vi "getDescription.vi"(8 "error in (no error)":errorcluster, 11 "Milk in":refnum<class "Milk.lvclass">) -> (0 "error out":errorcluster, 2 "description":string, 3 "Milk out":refnum<class "Milk.lvclass">)   [LabVIEW 2013, in "Milk.lvclass"]
uses:
  Milk.lvclass
  Milk.lvclass/Milk.ctl
  Beverage/Beverage.lvclass
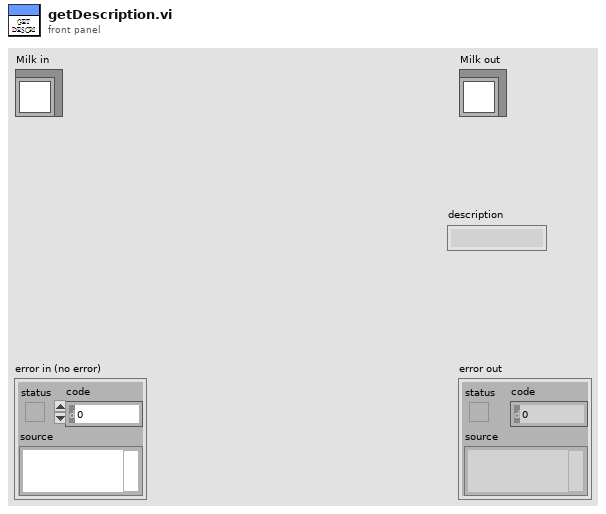
[diagram p1: front panel]
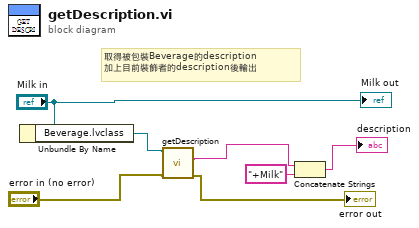
[diagram p0: block diagram]
diagram:
  # "取得被包裝Beverage的description\n加上目前裝飾者的description後輸出"
  n1 = Unbundle By Name("Milk in") -> ("Beverage.lvclass"=w4:refnum<class "Beverage.lvclass">)
  n2 = call-dynamic "getDescription.vi"("error in (no error)"="error in (no error)", "Beverage in"=w4) -> ("error out"=→"error out":errorcluster, "description"=w1:string)  [unwired: 7 in, 1 out]
  n3 = Concatenate Strings(w1, "+Milk" ("description")) -> (→"description":string)
  "Milk out" <- "Milk in"
